vi "Core.vi"() -> ()   [LabVIEW 2018]
uses:
  Message Class/Message.lvclass
  Message Class/Ini/Initialise.lvclass
  F:/Gitlab Repository/LabVIEW-Study/2.Deriving the Actor Core in Actor Framework/Lv2018/Message Class/Message.lvclass
  Standard Class/Standard.lvclass
  F:/Gitlab Repository/LabVIEW-Study/2.Deriving the Actor Core in Actor Framework/Lv2018/Counter Class/Counter.lvclass
  Complex Class/Complex.lvclass
  Message Class/Increment/Increment.lvclass
  Message Class/Stop/Stop.lvclass
  Counter Class/Counter.lvclass
panel:
  out "Current Count":cdb
  in  "Complex":bool
  in  "Increment":bool
  in  "Stop":bool
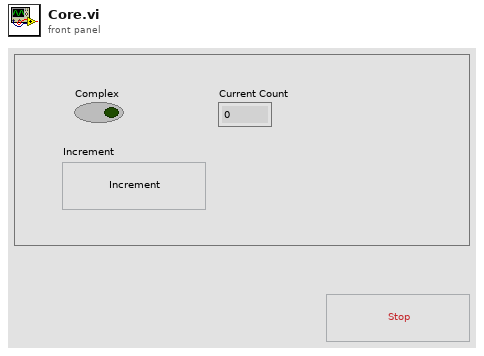
[diagram p1: front panel]
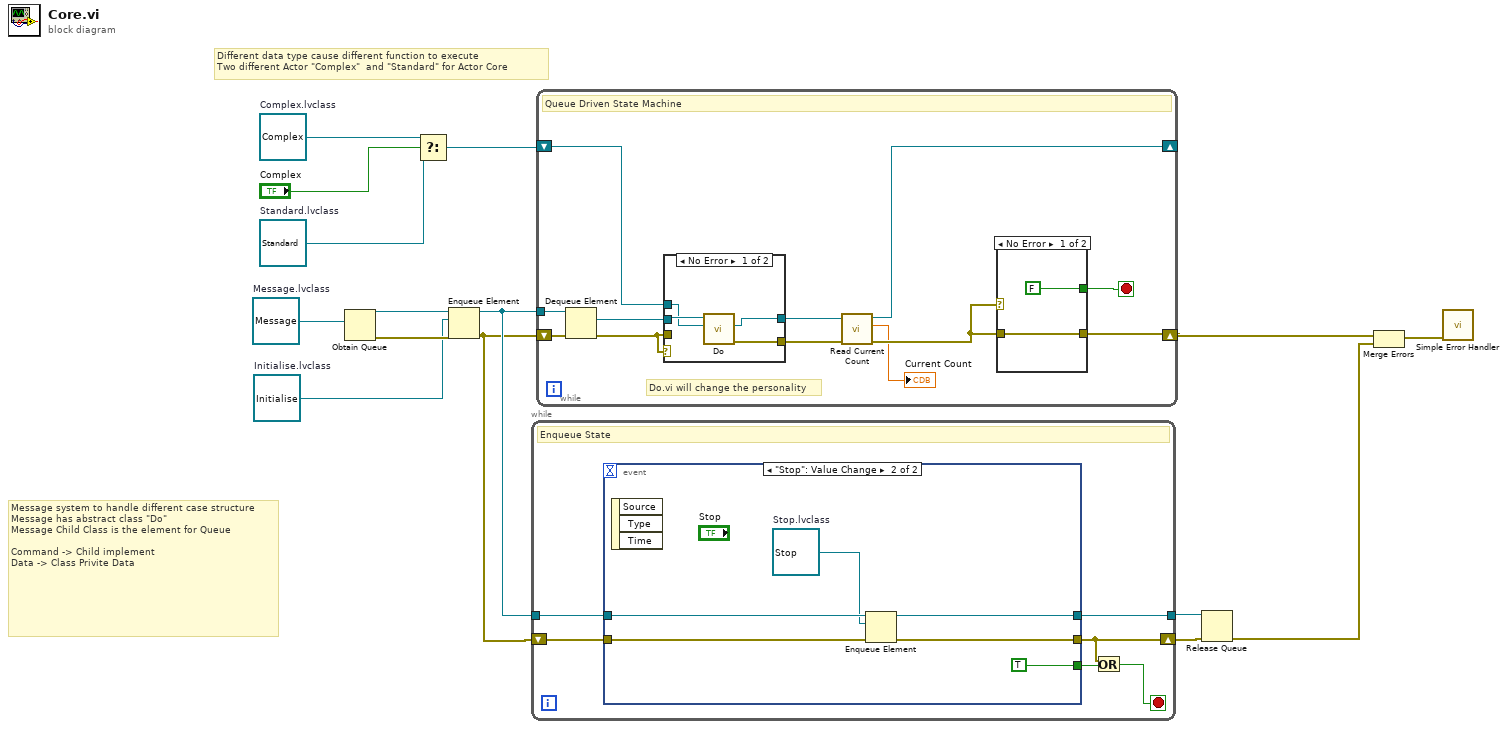
[diagram p0: block diagram]
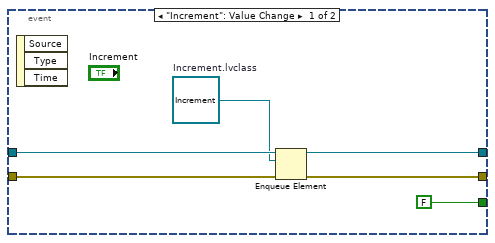
[diagram p2: hidden frame]
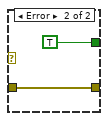
[diagram p3: hidden frame]
diagram:
  w2 = refnum<class "Complex.lvclass"> refnum  # Complex.lvclass
  w3 = refnum<class "Standard.lvclass"> refnum  # Standard.lvclass
  w9 = refnum<class "Initialise.lvclass"> refnum  # Initialise.lvclass
  w10 = refnum<class "Message.lvclass"> refnum  # Message.lvclass
  # "Message system to handle different case structure \nMessage has abstract class \"Do\"\nMessage Child Class is the element for Queue\n\nCommand -> Child implement \nData -> Class Privite Data"
  # "Different data type cause different function to execute \nTwo different Actor \"Complex\"  and \"Standard\" for Actor Core"
  n1 = Obtain Queue(element data type=w10) -> (queue out=w15:refnum<queue>, error out=w14:errorcluster)  [unwired: 4 in, 1 out]
  n2 = Select(t=w2, s="Complex", f=w3) -> (s? t:f=w1:refnum<class "Counter.lvclass">)
  n3 = Enqueue Element(queue=w15, element=w9, error in (no error)=w14) -> (queue out=w13:refnum<queue>, error out=w12:errorcluster)  [unwired: 1 in, 1 out]
  n4 = while {
    tunnel: w13 -> [w21]
    shift-right: [w19] -> w7
    shift-left: w12 -> [w20]
    tunnel: [w16] -> w6
    stop <- w17 stop-if-true
    # "Enqueue State"
    n5 = event shown="[1] \"Stop\": Value Change" {
      selector: _ -> [_ _]
      dyn-events: _ -> [_ _]
      timeout: _ -> [_ _]
      tunnel: w21 -> [w27 w33]
      tunnel: w20 -> [w26 w32]
      tunnel: [w25 w31] -> w19
      tunnel: [FALSE TRUE] -> w18
      tunnel: [w22 w28] -> w16
      event "Increment": Value Change {
        w23 = refnum<class "Increment.lvclass"> refnum  # Increment.lvclass
        n6 = event-data() -> ()  [unwired: 1 in, 3 out]
        n7 = Enqueue Element(queue=w27, element=w23, error in (no error)=w26) -> (queue out=w22:refnum<queue>, error out=w25:errorcluster)  [unwired: 1 in, 1 out]
      }
      event "Stop": Value Change {
        w29 = refnum<class "Stop.lvclass"> refnum  # Stop.lvclass
        n8 = event-data() -> ()  [unwired: 1 in, 3 out]
        n9 = Enqueue Element(queue=w33, element=w29, error in (no error)=w32) -> (queue out=w28:refnum<queue>, error out=w31:errorcluster)  [unwired: 1 in, 1 out]
      }
    }
    n10 = Or(x=w19, y=w18) -> (x .or. y?=w17:bool)
  }
  n11 = while {
    tunnel: w13 -> [w44]
    shift-right: [w41] -> w11
    shift-left: w12 -> [w45]
    shift-right: [w36] -> _
    shift-left: w1 -> [w34]
    stop <- w40 stop-if-true
    # "Do.vi will change the personality"
    # "Queue Driven State Machine"
    n12 = Dequeue Element(queue=w44, error in (no error)=w45) -> (element=w43:refnum<class "Message.lvclass">, error out=w42:errorcluster)  [unwired: 1 in, 2 out]
    n13 = case shown="No Error" w42 {
      tunnel: w43 -> [w53 _]
      tunnel: w34 -> [w52 w54]
      tunnel: [w51 w54] -> w39
      tunnel: [w50 w55] -> w38
      tunnel: w42 -> [_ w55]
      frame No Error {
        n14 = call-dynamic "Do.vi"("Counter In"=w52, "Message in"=w53) -> ("error out"=w50:errorcluster, "Counter Out"=w51:refnum<class "Counter.lvclass">)  [unwired: 7 in, 1 out]
      }
      frame Error {
      }
    }
    n15 = call-dynamic "Read Current Count.vi"("error in (no error)"=w38, "Counter in"=w39) -> ("error out"=w37:errorcluster, "Current Count"=→"Current Count":cdb, "Counter out"=w36:refnum<class "Counter.lvclass">)  [unwired: 7 in]
    n16 = case shown="No Error" w37 {
      tunnel: w37 -> [w47 w49]
      tunnel: [w47 w49] -> w41
      tunnel: [FALSE TRUE] -> w40
      frame No Error {
      }
      frame Error {
      }
    }
  }
  n17 = Release Queue(queue=w6, error in (no error)=w7) -> (error out=w5:errorcluster)  [unwired: 1 in, 2 out]
  n18 = Merge Errors(w11, w5) -> (w8:errorcluster)
  n19 = call <vilib>:"Simple Error Handler.vi"("error in (no error)"=w8) -> ()  [unwired: 4 in, 5 out]
